vi "collatzStep.vi"(10 "gradn":u64) -> (2 "gradnext":u64)   [LabVIEW 2024]
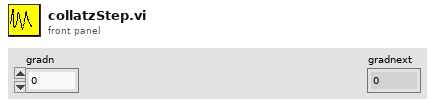
[diagram p1: front panel]
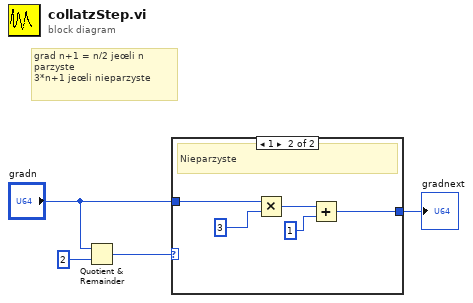
[diagram p0: block diagram]
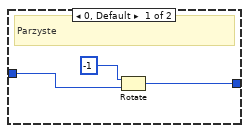
[diagram p2: hidden frame]
diagram:
  # "grad n+1 = n/2 jeœli n parzyste\n3*n+1 jeœli nieparzyste"
  n1 = Quotient & Remainder(x="gradn", y=2) -> (x-y*floor(x/y)=w3:u64)  [unwired: 1 out]
  n2 = case shown="1" w3 {
    tunnel: "gradn" -> [w6 w11]
    tunnel: [w5 w8] -> w1
    frame 0, Default {
      # "Parzyste"
      n3 = Rotate(1:w6, 2:-1) -> (0:w5:u64)
    }
    frame 1 {
      # "Nieparzyste"
      n4 = Multiply(x=w11, y=3) -> (x*y=w10:u64)
      n5 = Add(x=w10, y=1) -> (x+y=w8:u64)
    }
  }
  "gradnext" <- w1
